vi "test12-RegisterMultipleStatesToOneState.vi"(8 "error in (no error)":errorcluster, 11 "TestCase in":refnum<class "testcase-CSMBroadcast.lvclass">) -> (0 "error out":errorcluster, 3 "TestCase out":refnum<class "testcase-CSMBroadcast.lvclass">)   [LabVIEW 2017, in "testcase-CSMBroadcast.lvclass"]
uses:
  testcase-CSMBroadcast.lvclass
  e86cc395-d992-44ca-a767-e0e34a6869d5.vi
  3bcad317-1b89-4687-aa9b-3ccbe7d60bbb.vi
  2694ea11-6498-4afa-8b48-991e2fec04f6.vi
  src/user.lib/_NEVSTOP/Communicable State Machine(CSM)/AdvanceAPI/CSM - Revert Arguments-Safe String.vi
  src/user.lib/_NEVSTOP/Communicable State Machine(CSM)/AdvanceAPI/CSM - Make String Arguments Safe.vi
  src/user.lib/_NEVSTOP/Communicable State Machine(CSM)/AdvanceAPI/CSM - Break Down Multiple States String.vi
  src/user.lib/_NEVSTOP/Communicable State Machine(CSM)/AdvanceAPI/CSM - Compact Multiple States.vi
  src/user.lib/_NEVSTOP/Communicable State Machine(CSM)/AdvanceAPI/CSM - Keywords.vi
  src/user.lib/_NEVSTOP/Communicable State Machine(CSM)/_Polymophic/CSM - Replace Marks in Messages.vi
  src/user.lib/_NEVSTOP/Communicable State Machine(CSM)/_Shared/Trim Single-line Text.vi
  src/user.lib/_NEVSTOP/Communicable State Machine(CSM)/AdvanceAPI/CSM - Set Module Attribute.vi
  src/user.lib/_NEVSTOP/Communicable State Machine(CSM)/AdvanceAPI/CSM - Get Module Attribute.vi
  <vilib>/addons/_JKI Toolkits/VI Tester/TestCase.llb/TestCase.lvclass
  src/user.lib/_NEVSTOP/Communicable State Machine(CSM)/Communicable State Machine.lvlib
  C:/Program Files (x86)/National Instruments/LabVIEW 2017/vi.lib/addons/_JKI Toolkits/VI Tester/TestCase.llb/TestCase.lvclass
panel:
  out "LoopCount":i32
  out "State History":string
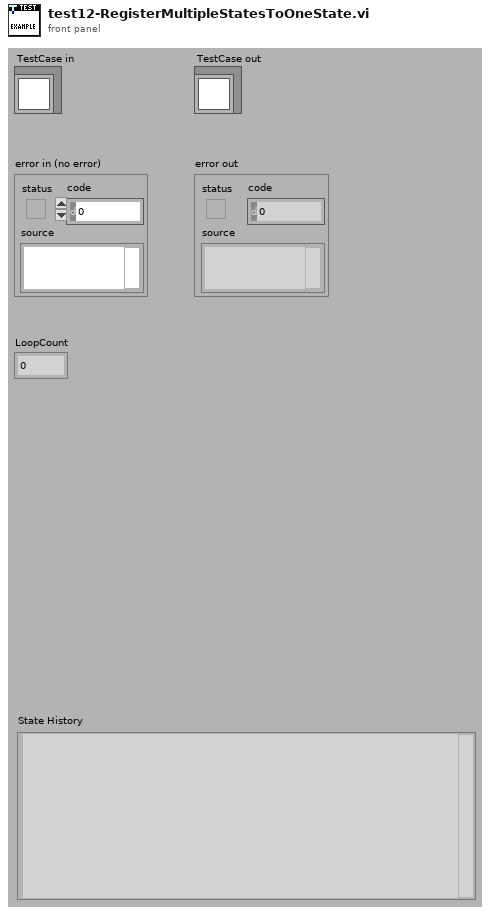
[diagram p1: front panel]
types:
  T1 = enum32{"Invalid", "Standard", "Closed", "Hidden", "Minimized", "Maximized"}
  T2 = enum32{"invalid app kind", "Development System", "Run Time System", "Student Edition", "Embedded LabVIEW", "Evaluation", "Custom"}
  T3 = typedef "Communicable State Machine.lvlib/_CSM_Response Source Message.ctl" = cluster{"‘State":string, "’Arguments":string, "’Error":errorcluster}
  T4 = cluster{"Current VI Reference":refnum<vi>, "Close Panel on Exit?":bool}
  T5 = cluster{"Core":cluster{"Current VI Reference":refnum<vi>, "Close Panel on Exit?":bool}, "Your Boolean data":bool, "Your string data":string, "TestData":i32}
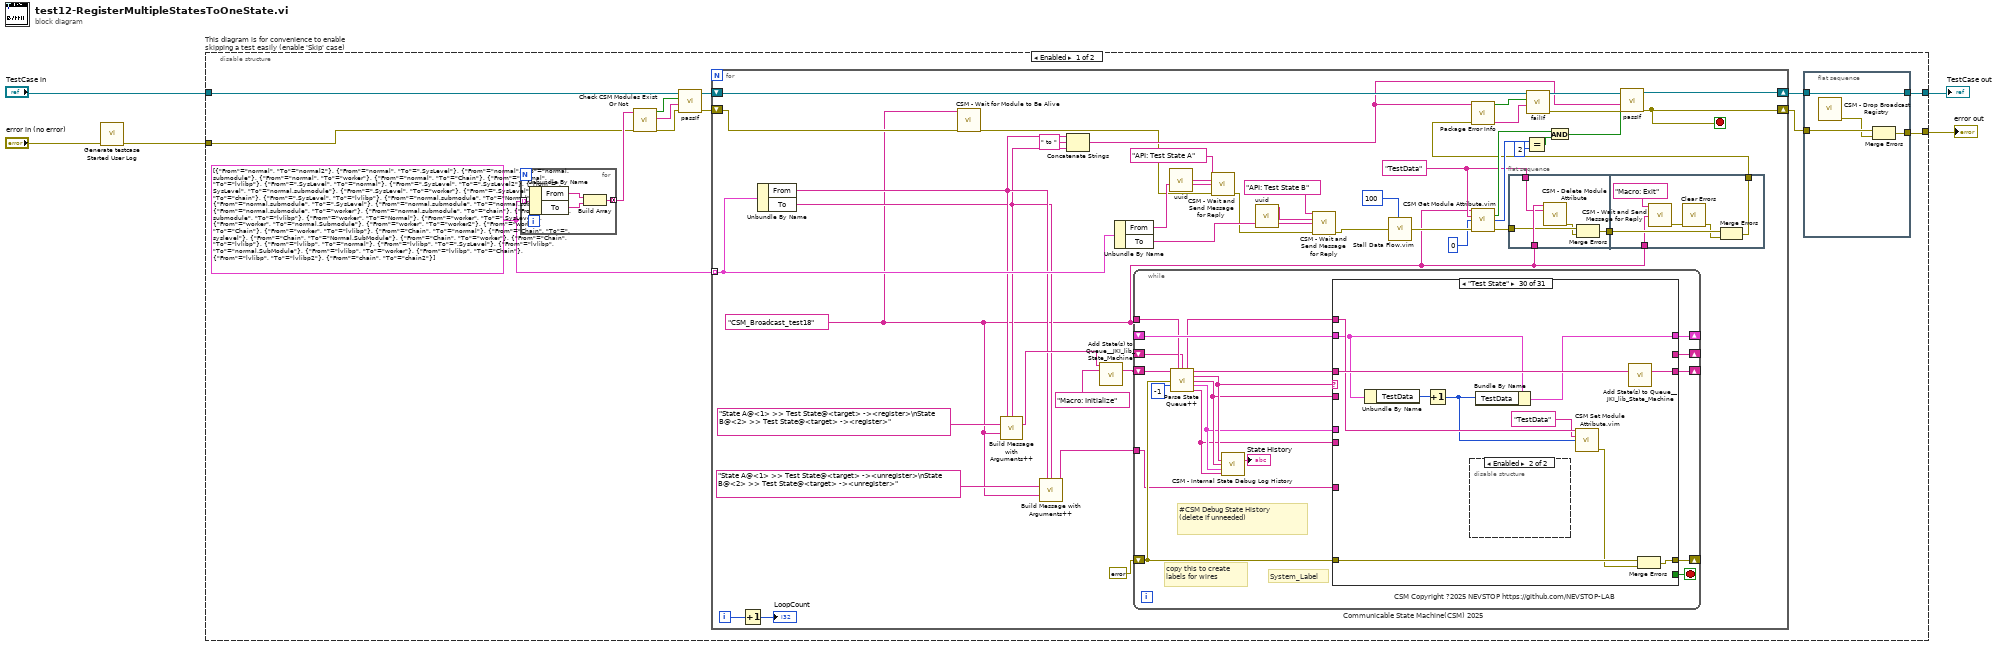
[diagram p0: block diagram]
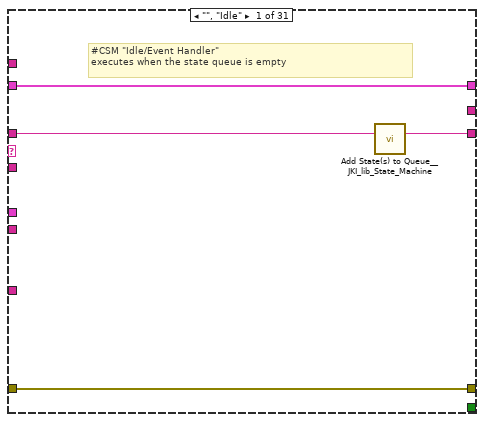
[diagram p2: hidden frame]
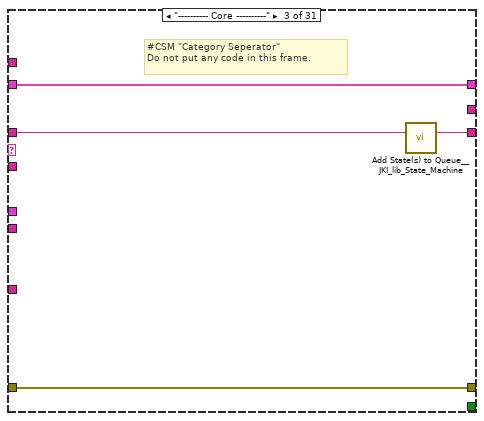
[diagram p4: hidden frame]
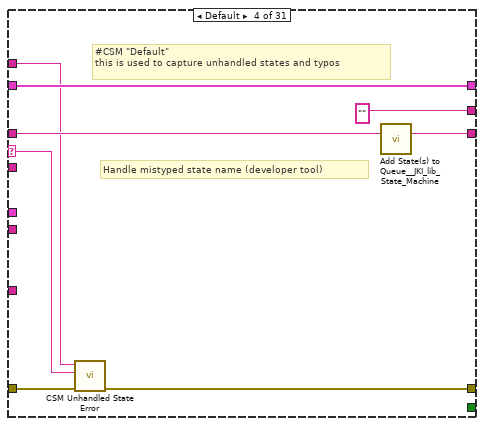
[diagram p5: hidden frame]
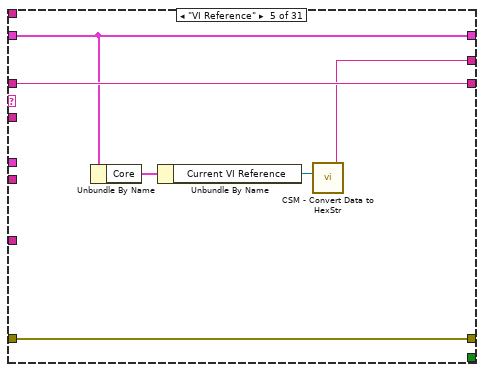
[diagram p6: hidden frame]
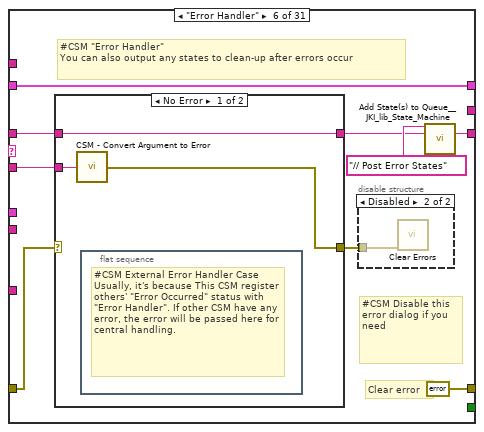
[diagram p7: hidden frame]
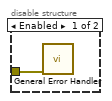
[diagram p8: hidden frame]
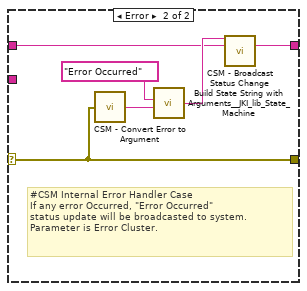
[diagram p9: hidden frame]
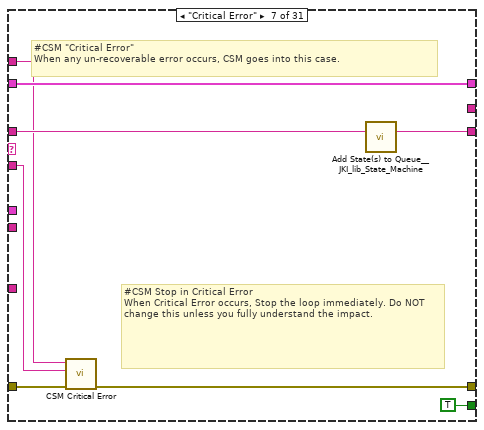
[diagram p10: hidden frame]
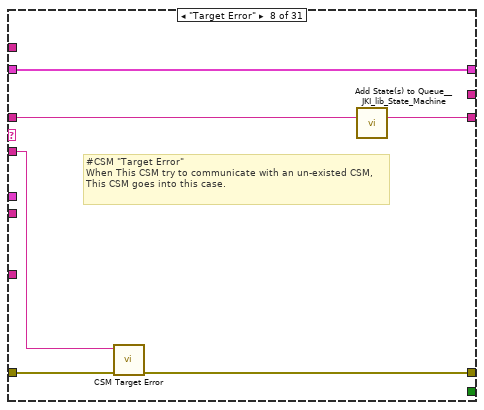
[diagram p11: hidden frame]
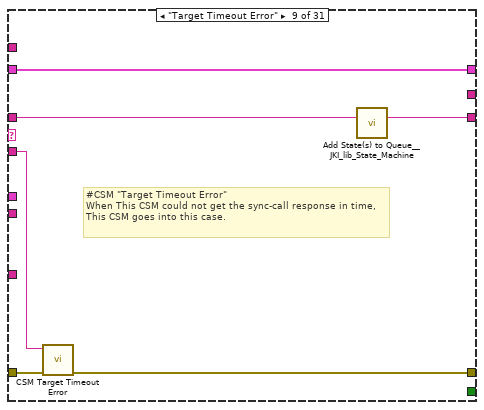
[diagram p12: hidden frame]
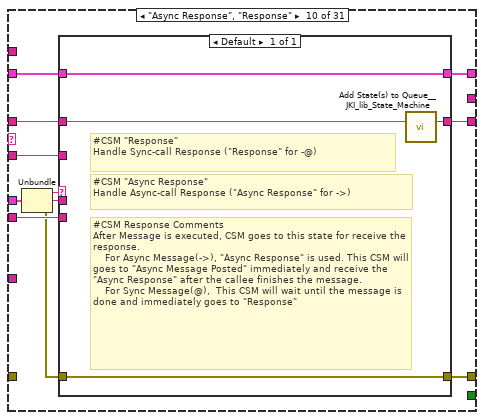
[diagram p13: hidden frame]
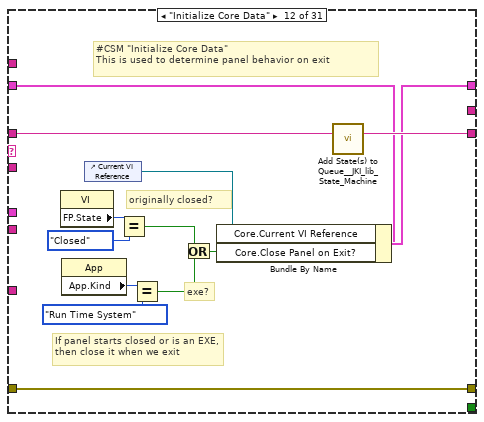
[diagram p15: hidden frame]
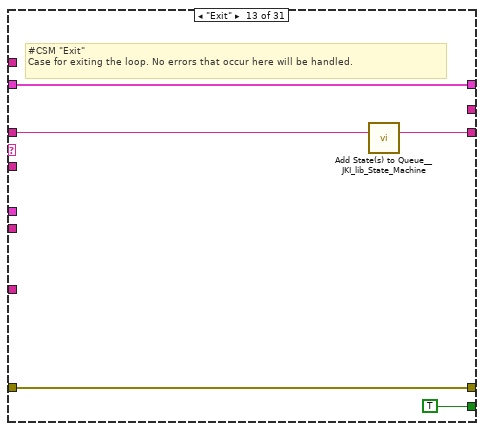
[diagram p16: hidden frame]
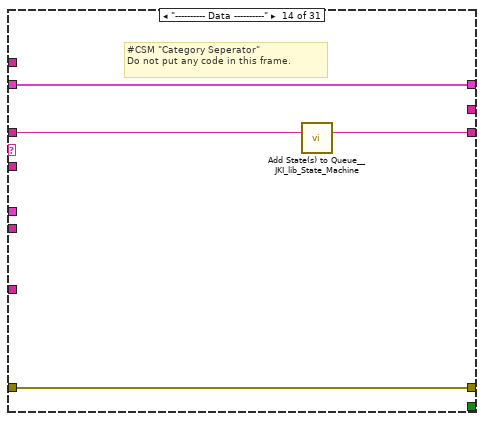
[diagram p17: hidden frame]
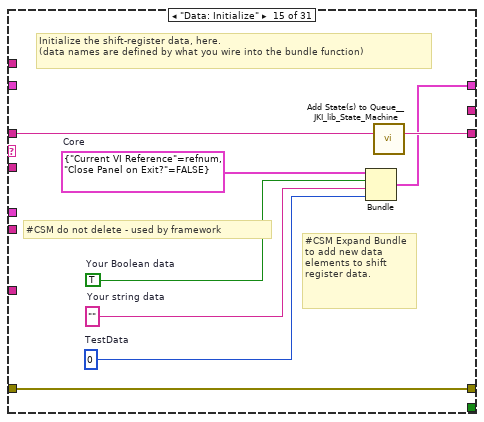
[diagram p18: hidden frame]
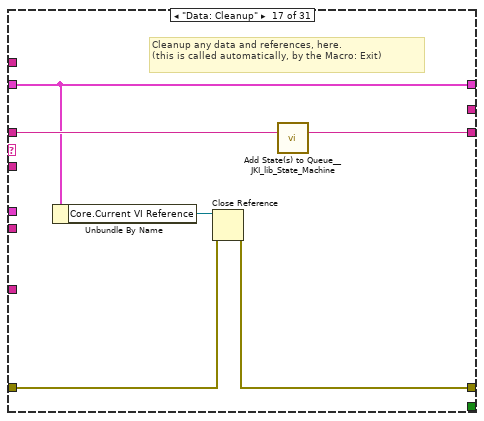
[diagram p20: hidden frame]
diagram:
  n1 = call "Generate testcase Started User Log.vi"("Error In"="error in (no error)") -> ("error out"=w1:errorcluster)  [unwired: 10 in]
  n2 = disable-structure "This diagram is for convenience to enable skipping a test easily (enable 'Skip' case)" shown="Enabled" {
    disable-tunnel: "TestCase in" -> [w9 w377]
    disable-tunnel: [w16 w375] -> w2
    disable-tunnel: [w15 w376] -> w4
    disable-tunnel: w1 -> [w6 w374]
    frame Enabled {
      w10 = cluster{"From":string, "To":string}[] [{"From"="normal", "To"="normal2"}, {"From"="normal", "To"=".SysLevel"}, {"From"="normal", "To"="normal.submodule"}, {"From"="normal", "To"="worker"}, {"From"="normal", "To"="Chain"}, {"From"="normal", "To"="lvlibp"}, {"From"=".SysLevel", "To"="normal"}, {"From"=".SysLevel", "To"=".SysLevel2"}, {"From"=".SysLevel", "To"="normal.submodule"}, {"From"=".SysLevel", "To"="worker"}, {"From"=".SysLevel", "To"="chain"}, {"From"=".SysLevel", "To"="lvlibp"}, {"From"="normal.submodule", "To"="Normal"}, {"From"="normal.submodule", "To"=".SysLevel"}, {"From"="normal.submodule", "To"="normal.submodule2"}, {"From"="normal.submodule", "To"="worker"}, {"From"="normal.submodule", "To"="chain"}, {"From"="normal.submodule", "To"="lvlibp"}, {"From"="worker", "To"="Normal"}, {"From"="worker", "To"=".SysLevel"}, {"From"="worker", "To"="normal.Submodule"}, {"From"="worker", "To"="worker2"}, {"From"="worker", "To"="Chain"}, {"From"="worker", "To"="lvlibp"}, {"From"="Chain", "To"="normal"}, {"From"="Chain", "To"=".syslevel"}, {"From"="Chain", "To"="Normal.SubModule"}, {"From"="Chain", "To"="worker"}, {"From"="Chain", "To"="lvlibp"}, {"From"="lvlibp", "To"="normal"}, {"From"="lvlibp", "To"=".SysLevel"}, {"From"="lvlibp", "To"="normal.SubModule"}, {"From"="lvlibp", "To"="worker"}, {"From"="lvlibp", "To"="Chain"}, {"From"="lvlibp", "To"="lvlibp2"}, {"From"="chain", "To"="chain2"}]
      n3 = for {
        tunnel: w10 -> [w22] mode=indexing
        tunnel: [w19] -> w13 mode=concatenating
        n4 = Unbundle By Name(w22) -> ("From"=w21:string, "To"=w20:string)
        n5 = Build Array(w21, w20) -> (w19:string[])
      }
      n6 = call "Check CSM Modules Exist Or Not.vi"("error in"=w6, "CSM names in"=w13) -> ("error out"=w11:errorcluster, "Debug string"=w12:string, "All Modules Exist?"=w14:bool)  [unwired: 7 in]
      n7 = call-dynamic "passIf.vi"("error in (no error)"=w11, "message (\"\")"=w12, "pass"=w14, "TestCase in"=w9) -> ("error out"=w7:errorcluster, "TestCase out"=w8:refnum<class "testcase-CSMBroadcast.lvclass">)  [unwired: 6 in]
      n8 = for {
        tunnel: w10 -> [w61] mode=indexing
        shift-right: [w48] -> w18
        shift-left: w8 -> [w39]
        shift-right: [w47] -> w17
        shift-left: w7 -> [w31]
        i -> [w46]
        stop <- w47 stop-if-true
        w50 = "TestData" ("Attribute")
        w29 = "CSM_Broadcast_test18" ("Name (\"\" to Use UUID)")
        n9 = Increment(x=w46) -> (x+1=→"LoopCount":i32)
        n10 = Unbundle By Name(w61) -> ("From"=w35:string, "To"=w34:string)
        n11 = call "CSM - Wait for Module to Be Alive.vi"("CSM Name"=w29, "error in (no error)"=w31) -> ("error out"=w30:errorcluster)  [unwired: 11 in, 2 out]
        n12 = call-poly "Build Message with Arguments++.vi"("States With Replace Token"="State A@<1> >> Test State@<target> -><register>\nState B@<2> >> Test State@<target> -><register>" ("Init State(\"Macro: Initialize\")"), "<target>"=w29, "<1>"=w35, "<2>"=w34) -> ("States"=w59:string)  [unwired: 11 in]
        n13 = call-poly "Build Message with Arguments++.vi"("States With Replace Token"="State A@<1> >> Test State@<target> -><unregister>\nState B@<2> >> Test State@<target> -><unregister>" ("Init State(\"Macro: Initialize\")"), "<target>"=w29, "<1>"=w35, "<2>"=w34) -> ("States"=w57:string)  [unwired: 11 in]
        n14 = Concatenate Strings(w35, " to " ("string"), w34) -> (w32:string)
        n15 = call <vilib>:"Add State(s) to Queue__JKI_lib_State_Machine.vi"("State(s) in Front (\"\")"=w59, "State(s) in (\"\")"="Macro: Initialize" ("Init State(\"Macro: Initialize\")")) -> ("States Out"=w62:string)  [unwired: 13 in]
        n16 = Unbundle By Name(w61) -> ("From"=w68:string, "To"=w67:string)
        n17 = while "Communicable State Machine(CSM) 2025" {
          shift-right: [w95] -> _
          shift-left: _ -> [w94]
          shift-right: [w98] -> _
          shift-left: errorcluster {"status"=FALSE, "code"=0, "source"=""} ("error out") -> [w93]
          shift-right: [w97] -> _
          shift-left: w62 -> [w99]
          tunnel: w29 -> [w91]
          shift-right: [w92] -> _
          shift-left: _ -> [w85]
          tunnel: w57 -> [w82]
          stop <- w96 stop-if-true
          # "#CSM Debug State History\n(delete if unneeded)"
          # "copy this to create labels for wires"
          # "System_Label"
          # "CSM Copyright ?2025 NEVSTOP https://github.com/NEVSTOP-LAB"
          n18 = call "Parse State Queue++.vi"("State Queue"=w99, "Name (\"\" to Use UUID)"=w91, "Response Arguments"=w85, "Previous Error"=w93, "Dequeue (1 ms)"=-1 ("Timeout")) -> ("Name Used"=w86:string, "Remaining States"=w100:string, "Current State"=w90:string, "Arguments"=w89:string, "Additional Information"=w88:T3, "Source CSM"=w87:string)  [unwired: 5 in]
          n19 = call "CSM - Internal State Debug Log History.vi"("State"=w90, "Arguments (\"\")"=w89, ">> Response Source Message >>"=w88, "Source (\"\")"=w87) -> ("Debug Log"=→"State History":string)  [unwired: 11 in]
          n20 = case shown="\"Test State\"" w90 {
            selector: w90 -> [_ _ _ w114 _ _ _ _ _ _ _ _ _ _ _ _ _ _ _ _ _ _ _ _ _ _ _ _ _ _ _]
            tunnel: w100 -> [w101 w106 w111 w118 w124 w130 w151 w157 w163 w171 w182 w196 w201 w205 w213 w215 w222 w226 w230 w236 w251 w320 w325 w333 w335 w339 w344 w351 w355 w366 w373]
            tunnel: w89 -> [_ _ _ _ _ w129 w147 w156 w161 w170 _ _ _ _ _ _ _ _ _ w231 w245 _ _ _ _ _ w342 _ _ _ _]
            tunnel: w94 -> [w102 w105 w108 w116 w123 w133 w152 w158 w164 w173 w181 w189 w199 w202 _ w214 w217 w223 w228 w234 w247 w317 w322 w330 w334 w338 w343 w348 w352 w358 w370]
            tunnel: [w103 w107 w109 w112 w125 errorcluster {"status"=FALSE, "code"=0, "source"=""} ("error out") w148 w154 w160 w176 w183 w193 w198 w203 w210 w216 w218 w224 w227 w232 w248 w318 w323 w331 w336 w340 w345 w349 w353 w360 w371] -> w98
            tunnel: w93 -> [w103 w107 w109 w119 w125 w131 w153 w155 w162 _ w183 w193 w198 w203 w210 w216 w219 w224 w227 w233 w249 w318 w323 w331 w336 w340 w345 w349 w353 w364 w371]
            tunnel: [w104 w106 w110 w117 w124 w126 w150 w159 w165 w172 w182 w195 w200 w204 w212 w215 w221 w225 w229 w235 w250 w319 w324 w332 w335 w339 w344 w350 w354 w365 w372] -> w97
            tunnel: [_ _ _ _ _ _ TRUE _ _ _ _ _ TRUE _ _ _ _ _ _ _ _ _ _ _ _ _ _ _ _ _ _] -> w96
            tunnel: [w102 w105 w108 w116 w123 w133 w152 w158 w164 w174 w181 w194 w199 w202 w211 w214 w217 w223 w228 w234 w247 w317 w322 w330 w334 w338 w343 w348 w352 w362 w370] -> w95
            tunnel: w87 -> [_ _ _ _ _ _ _ _ _ w168 _ _ _ _ _ _ _ _ _ _ _ _ _ _ _ _ _ _ _ _ _]
            tunnel: w88 -> [_ _ _ _ _ _ _ _ _ w175 _ _ _ _ _ _ _ _ _ _ _ _ _ _ _ _ _ _ _ _ _]
            tunnel: [_ _ _ "" w120 _ _ _ _ _ _ _ _ _ _ _ _ _ _ _ _ _ _ _ _ "API1 Response" w341 _ _ _ _] -> w92
            tunnel: w86 -> [_ _ _ w113 _ _ w146 _ _ _ _ _ _ _ _ _ _ _ _ _ _ _ _ _ _ _ _ _ _ w361 _]
            tunnel: w82 -> [_ _ _ _ _ _ _ _ _ _ _ _ _ _ _ _ _ _ _ _ _ _ _ w326 _ _ _ _ _ _ _]
            frame "", "Idle" {
              # "#CSM \"Idle/Event Handler\"\nexecutes when the state queue is empty"
              n21 = call <vilib>:"Add State(s) to Queue__JKI_lib_State_Machine.vi"("State(s) in (\"\")"=w101) -> ("States Out"=w104:string)  [unwired: 14 in]
            }
            frame "CSM Documentation" {
              # "#CSM README FIRST\n\nCommunicable State Machine(CSM) is a LabVIEW application framework that builds upon JKI State Machine(JKISM). It follows the pattern of JKISM and extends the keywords to describe message communication between modules, including concepts such as Sync-Message, Async-Message, Subscription/Unsubscription of status - essential elements for creating reusable code modules. For more information, please visit the CSM wiki: https://nevstop-lab.github.io/CSM-Wiki/\n\nFor instructions on JKI State Machine, visit: http://jki.net/state-machine/\nFor information about CSM, visit: https://github.com/NEVSTOP-LAB"
              # "#CSM \"Documentation\"\nCase for holding CSM Documenation"
            }
            frame "---------- Core ----------" {
              # "#CSM \"Category Seperator\"\nDo not put any code in this frame."
              n22 = call <vilib>:"Add State(s) to Queue__JKI_lib_State_Machine.vi"("State(s) in (\"\")"=w111) -> ("States Out"=w110:string)  [unwired: 14 in]
            }
            frame Default {
              # "#CSM \"Default\"\nthis is used to capture unhandled states and typos"
              # "Handle mistyped state name (developer tool)"
              n23 = call "CSM Unhandled State Error.vi"("error in (no error)"=w119, "Undefined State"=w114, "CSM Name"=w113) -> ("error out"=w112:errorcluster)  [unwired: 8 in]
              n24 = call <vilib>:"Add State(s) to Queue__JKI_lib_State_Machine.vi"("State(s) in (\"\")"=w118) -> ("States Out"=w117:string)  [unwired: 14 in]
            }
            frame "VI Reference" {
              n25 = Unbundle By Name(w123) -> ("Core"=w122:T4)
              n26 = Unbundle By Name(w122) -> ("Current VI Reference"=w121:refnum<vi>)
              n27 = call "CSM - Convert Data to HexStr.vi"("Variant"=w121) -> ("HEX String (0-9,A-F)"=w120:string)  [unwired: 8 in]
            }
            frame "Error Handler" {
              # "#CSM Disable this error dialog if you need"
              # "#CSM \"Error Handler\"\nYou can also output any states to clean-up after errors occur"
              # "Clear error"
              n28 = case shown="No Error" w131 {
                selector: w131 -> [_ w140]
                tunnel: [w139 w142] -> w127
                tunnel: w130 -> [w139 w141]
                tunnel: w129 -> [w138 _]
                tunnel: [w137 w140] -> w132
                frame No Error {
                  n29 = call "CSM - Convert Argument to Error.vi"("Argument"=w138) -> ("Error"=w137:errorcluster)  [unwired: 4 in]
                  n30 = flat-sequence {
                    frame #0 {
                      # "#CSM External Error Handler Case\nUsually, it's because This CSM register others' \"Error Occurred\" status with \"Error Handler\". If other CSM have any error, the error will be passed here for central handling."
                    }
                  }
                }
                frame Error {
                  # "#CSM Internal Error Handler Case \nIf any error Occurred, \"Error Occurred\" \nstatus update will be broadcasted to system.\nParameter is Error Cluster."
                  n31 = call "CSM - Convert Error to Argument.vi"("Error"=w140) -> ("Argument"=w144:string)  [unwired: 4 in]
                  n32 = call <vilib>:"Build State String with Arguments__JKI_lib_State_Machine.vi"("Arguments (\"\")"=w144, "State"="Error Occurred" ("Status with Arguments")) -> ("State with Arguments"=w143:string)  [unwired: 4 in]
                  n33 = call "CSM - Broadcast Status Change.vi"("Status With Arguments"=w143, "State Queue"=w141) -> ("Remaining States"=w142:string)  [unwired: 13 in]
                }
              }
              n34 = disable-structure shown="Disabled" {
                disable-tunnel: w132 -> [w135 w136]
                frame Enabled {
                  n35 = call <vilib>:"General Error Handler.vi"("error in (no error)"=w135) -> ()  [unwired: 10 in, 5 out]
                }
                frame Disabled {
                  n36 = call <vilib>:"Clear Errors.vi"("error in (no error)"=w136) -> ()  [unwired: 5 in, 2 out]
                }
              }
              n37 = call <vilib>:"Add State(s) to Queue__JKI_lib_State_Machine.vi"("State(s) in Front (\"\")"="// Post Error States", "State(s) in (\"\")"=w127) -> ("States Out"=w126:string)  [unwired: 13 in]
            }
            frame "Critical Error" {
              # "#CSM Stop in Critical Error\nWhen Critical Error occurs, Stop the loop immediately. Do NOT change this unless you fully understand the impact."
              # "#CSM \"Critical Error\"\nWhen any un-recoverable error occurs, CSM goes into this case."
              n38 = call "CSM Critical Error.vi"("error in (no error)"=w153, "Arugments (As Reason)"=w147, "CSM Name"=w146) -> ("error out"=w148:errorcluster)  [unwired: 8 in]
              n39 = call <vilib>:"Add State(s) to Queue__JKI_lib_State_Machine.vi"("State(s) in (\"\")"=w151) -> ("States Out"=w150:string)  [unwired: 14 in]
            }
            frame "Target Error" {
              # "#CSM \"Target Error\"\nWhen This CSM try to communicate with an un-existed CSM, This CSM goes into this case."
              n40 = call "CSM Target Error.vi"("error in (no error)"=w155, "Arguments (As CSM Name)"=w156) -> ("error out"=w154:errorcluster)  [unwired: 9 in]
              n41 = call <vilib>:"Add State(s) to Queue__JKI_lib_State_Machine.vi"("State(s) in (\"\")"=w157) -> ("States Out"=w159:string)  [unwired: 14 in]
            }
            frame "Target Timeout Error" {
              # "#CSM \"Target Timeout Error\"\nWhen This CSM could not get the sync-call response in time, This CSM goes into this case."
              n42 = call "CSM Target Timeout Error.vi"("error in (no error)"=w162, "Arguments (As CSM Name)"=w161) -> ("error out"=w160:errorcluster)  [unwired: 9 in]
              n43 = call <vilib>:"Add State(s) to Queue__JKI_lib_State_Machine.vi"("State(s) in (\"\")"=w163) -> ("States Out"=w165:string)  [unwired: 14 in]
            }
            frame "Async Response", "Response" {
              n44 = Unbundle(w175) -> ("‘State"=w169:string, "’Arguments"=w167:string, "’Error"=w166:errorcluster)
              n45 = case shown="Default" w169 {
                tunnel: [w180] -> w176
                tunnel: w166 -> [w180]
                tunnel: [w179] -> w174
                tunnel: w173 -> [w179]
                tunnel: [w177] -> w172
                tunnel: w171 -> [w178]
                tunnel: w170 -> [_]
                tunnel: w168 -> [_]
                tunnel: w167 -> [_]
                frame Default {
                  # "#CSM Response Comments\nAfter Message is executed, CSM goes to this state for receive the response.\n    For Async Message(->), \"Async Response\" is used. This CSM will goes to \"Async Message Posted\" immediately and receive the \"Async Response\" after the callee finishes the message.\n    For Sync Message(@),  This CSM will wait until the message is done and immediately goes to \"Response\""
                  # "#CSM \"Async Response\"\nHandle Async-call Response (\"Async Response\" for ->)"
                  # "#CSM \"Response\"\nHandle Sync-call Response (\"Response\" for -@)"
                  n46 = call <vilib>:"Add State(s) to Queue__JKI_lib_State_Machine.vi"("State(s) in (\"\")"=w178) -> ("States Out"=w177:string)  [unwired: 14 in]
                }
              }
            }
            frame "Async Message Posted" {
              # "#CSM \"Async Message Posted\"\nAfter Async Message is posted (-> or ->| ), CSM goes to this state for post-action.\nYou can use Argument - State to tell which Async Message is called."
            }
            frame "Initialize Core Data" {
              # "#CSM \"Initialize Core Data\"\nThis is used to determine panel behavior on exit"
              # "originally closed?"
              # "exe?"
              # "If panel starts closed or is an EXE, then close it when we exit"
              n47 = property class="VI"() -> ("FP.State"=w186:T1)  [unwired: 2 in, 2 out]
              n48 = property class="App"() -> ("App.Kind"=w192:T2)  [unwired: 2 in, 2 out]
              n49 = control-ref of="Current VI Reference"() -> (w187:refnum<vi>)
              n50 = Equal?(x=w186, y=T1."Closed" ("Front Panel Window:State")) -> (x = y?=w184:bool)
              n51 = Equal?(x=w192, y=T2."Run Time System" ("Application:Kind")) -> (x = y?=w190:bool)
              n52 = Or(x=w184, y=w190) -> (x .or. y?=w188:bool)
              n53 = Bundle By Name(cluster=w189, "Core.Current VI Reference"=w187, "Core.Close Panel on Exit?"=w188) -> (w194:T5)
              n54 = call <vilib>:"Add State(s) to Queue__JKI_lib_State_Machine.vi"("State(s) in (\"\")"=w196) -> ("States Out"=w195:string)  [unwired: 14 in]
            }
            frame "Exit" {
              # "#CSM \"Exit\"\nCase for exiting the loop. No errors that occur here will be handled."
              n55 = call <vilib>:"Add State(s) to Queue__JKI_lib_State_Machine.vi"("State(s) in (\"\")"=w201) -> ("States Out"=w200:string)  [unwired: 14 in]
            }
            frame "---------- Data ----------" {
              # "#CSM \"Category Seperator\"\nDo not put any code in this frame."
              n56 = call <vilib>:"Add State(s) to Queue__JKI_lib_State_Machine.vi"("State(s) in (\"\")"=w205) -> ("States Out"=w204:string)  [unwired: 14 in]
            }
            frame "Data: Initialize" {
              w206 = 0  # TestData
              w207 = T4 {"Current VI Reference"=refnum, "Close Panel on Exit?"=FALSE}  # Core
              w209 = TRUE  # Your Boolean data
              w208 = ""  # Your string data
              # "#CSM do not delete - used by framework"
              # "#CSM Expand Bundle to add new data elements to shift register data."
              # "Initialize the shift-register data, here.\n(data names are defined by what you wire into the bundle function)"
              n57 = Bundle("Core"=w207, "Your Boolean data"=w209, "Your string data"=w208, "TestData"=w206) -> (w211:T5)  [unwired: 1 in]
              n58 = call <vilib>:"Add State(s) to Queue__JKI_lib_State_Machine.vi"("State(s) in (\"\")"=w213) -> ("States Out"=w212:string)  [unwired: 14 in]
            }
            frame "Data: Update Indicators" {
            }
            frame "Data: Cleanup" {
              # "Cleanup any data and references, here.\n(this is called automatically, by the Macro: Exit)"
              n59 = Unbundle By Name(w217) -> ("Core.Current VI Reference"=w220:refnum<vi>)
              n60 = Close Reference(reference=w220, error in (no error)=w219) -> (error out=w218:errorcluster)
              n61 = call <vilib>:"Add State(s) to Queue__JKI_lib_State_Machine.vi"("State(s) in (\"\")"=w222) -> ("States Out"=w221:string)  [unwired: 14 in]
            }
            frame "---------- UI ----------" {
              # "#CSM \"Category Seperator\"\nDo not put any code in this frame."
              n62 = call <vilib>:"Add State(s) to Queue__JKI_lib_State_Machine.vi"("State(s) in (\"\")"=w226) -> ("States Out"=w225:string)  [unwired: 14 in]
            }
            frame "UI: Initialize" {
              # "#CSM \"UI: Initialize\"\nInitialize the User Interface, here.\n(this is called automatically, by the Macro: Init)"
              n63 = call <vilib>:"Add State(s) to Queue__JKI_lib_State_Machine.vi"("State(s) in (\"\")"=w230) -> ("States Out"=w229:string)  [unwired: 14 in]
            }
            frame "UI: Cursor Set" {
              # "#CSM \"UI: Cursor Set\"\nSet and Unset Cursor Busy.\n(Usage: \"UI: Cursor Set >> Busy|Idle\")"
              # "Argument"
              n64 = disable-structure shown="TARGET_TYPE!=Windows" {
                disable-tunnel: w233 -> [w239 w244]
                disable-tunnel: [w238 w244] -> w232
                disable-tunnel: w231 -> [w237 _]
                frame condition #0 (active) {
                  n65 = case shown="\"Idle\", Default" w237 {
                    tunnel: w239 -> [w241 w243]
                    tunnel: [w240 w242] -> w238
                    frame "Idle", Default {
                      n66 = call <vilib>:"Unset Busy.vi"("error in (no error)"=w241) -> ("error out"=w240:errorcluster)  [unwired: 10 in]
                    }
                    frame "Busy" {
                      n67 = call <vilib>:"Set Busy.vi"("error in (no error)"=w243) -> ("error out"=w242:errorcluster)  [unwired: 9 in, 1 out]
                    }
                  }
                }
                frame condition #1 {
                }
              }
              n68 = call <vilib>:"Add State(s) to Queue__JKI_lib_State_Machine.vi"("State(s) in (\"\")"=w236) -> ("States Out"=w235:string)  [unwired: 14 in]
            }
            frame "UI: Front Panel State" {
              # "#CSM \"UI: Front Panel State\"\nSet Front Panel Open or Closed\n(Usage: \"UI: Front Panel State >> Open|Close\")"
              # "Argument"
              n69 = Unbundle By Name(w247) -> ("Core.Current VI Reference"=w246:refnum<vi>)
              n70 = call <vilib>:"Add State(s) to Queue__JKI_lib_State_Machine.vi"("State(s) in (\"\")"=w251) -> ("States Out"=w250:string)  [unwired: 14 in]
              n71 = case shown="\"Close\", \"Closed\"" w245 {
                tunnel: w249 -> [w257 w272 w283 w296 w309]
                tunnel: [w259 w273 w285 w298 w311] -> w248
                tunnel: w246 -> [w258 w270 w284 w297 w310]
                frame "Open", "Standard", Default {
                  w252 = T1."Standard" ("State")
                  n72 = property class="VI"(reference=w258, error in=w257) -> (reference out=w255:refnum<vi>, error out=w256:errorcluster, "FP.State"=w254:T1)
                  n73 = Not Equal?(x=w254, y=w252) -> (x != y?=w253:bool)
                  n74 = case shown="True" w253 {
                    tunnel: [w263 w265] -> w259
                    tunnel: w256 -> [w262 w265]
                    tunnel: w255 -> [w261 _]
                    tunnel: w252 -> [w260 _]
                    frame True {
                      n75 = invoke class="VI" method="FP.Open"(reference=w261, error in=w262, "Activate"=TRUE, "State"=w260) -> (error out=w263:errorcluster)  [unwired: 1 in, 4 out]
                    }
                    frame False {
                    }
                  }
                }
                frame "Close", "Closed" {
                  n76 = property class="VI"(reference=w270, error in=w272) -> (reference out=w269:refnum<vi>, error out=w271:errorcluster, "FP.State"=w267:T1)
                  n77 = Not Equal?(x=w267, y=T1."Closed" ("Front Panel Window:State")) -> (x != y?=w266:bool)
                  n78 = case shown="False" w266 {
                    tunnel: [w274 w277] -> w273
                    tunnel: w271 -> [w274 w276]
                    tunnel: w269 -> [_ w275]
                    frame False {
                    }
                    frame True {
                      n79 = invoke class="VI" method="FP.Close"(reference=w275, error in=w276) -> (error out=w277:errorcluster)  [unwired: 1 in, 2 out]
                    }
                  }
                }
                frame "Hidden", "Hide" {
                  w278 = T1."Hidden" ("State")
                  n80 = property class="VI"(reference=w284, error in=w283) -> (reference out=w281:refnum<vi>, error out=w282:errorcluster, "FP.State"=w280:T1)
                  n81 = Not Equal?(x=w280, y=w278) -> (x != y?=w279:bool)
                  n82 = case shown="True" w279 {
                    tunnel: [w289 w290] -> w285
                    tunnel: w282 -> [w288 w290]
                    tunnel: w281 -> [w287 _]
                    tunnel: w278 -> [w286 _]
                    frame True {
                      n83 = invoke class="VI" method="FP.Open"(reference=w287, error in=w288, "State"=w286) -> (error out=w289:errorcluster)  [unwired: 2 in, 4 out]
                    }
                    frame False {
                    }
                  }
                }
                frame "Minimize", "Minimized" {
                  w291 = T1."Minimized" ("State")
                  n84 = property class="VI"(reference=w297, error in=w296) -> (reference out=w294:refnum<vi>, error out=w295:errorcluster, "FP.State"=w293:T1)
                  n85 = Not Equal?(x=w293, y=w291) -> (x != y?=w292:bool)
                  n86 = case shown="True" w292 {
                    tunnel: [w302 w303] -> w298
                    tunnel: w295 -> [w301 w303]
                    tunnel: w294 -> [w300 _]
                    tunnel: w291 -> [w299 _]
                    frame True {
                      n87 = invoke class="VI" method="FP.Open"(reference=w300, error in=w301, "State"=w299) -> (error out=w302:errorcluster)  [unwired: 2 in, 4 out]
                    }
                    frame False {
                    }
                  }
                }
                frame "Maximize", "Maximized" {
                  w304 = T1."Maximized" ("State")
                  n88 = property class="VI"(reference=w310, error in=w309) -> (reference out=w307:refnum<vi>, error out=w308:errorcluster, "FP.State"=w306:T1)
                  n89 = Not Equal?(x=w306, y=w304) -> (x != y?=w305:bool)
                  n90 = case shown="True" w305 {
                    tunnel: [w315 w316] -> w311
                    tunnel: w308 -> [w314 w316]
                    tunnel: w307 -> [w313 _]
                    tunnel: w304 -> [w312 _]
                    frame True {
                      n91 = invoke class="VI" method="FP.Open"(reference=w313, error in=w314, "State"=w312) -> (error out=w315:errorcluster)  [unwired: 2 in, 4 out]
                    }
                    frame False {
                    }
                  }
                }
              }
            }
            frame "---------- Macro ----------" {
              # "#CSM \"Category Seperator\"\nDo not put any code in this frame."
              n92 = call <vilib>:"Add State(s) to Queue__JKI_lib_State_Machine.vi"("State(s) in (\"\")"=w320) -> ("States Out"=w319:string)  [unwired: 14 in]
            }
            frame "Macro: Initialize" {
              # "#CSM \"Macro: Initialize\"\nInitialization Macro (This is called once, when the VI starts)"
              n93 = call <vilib>:"Add State(s) to Queue__JKI_lib_State_Machine.vi"("State(s) in Front (\"\")"="Data: Initialize\nInitialize Core Data\nData: Update Indicators", "State(s) in (\"\")"=w325) -> ("States Out"=w324:string)  [unwired: 13 in]
            }
            frame "Macro: Exit" {
              # "#CSM \"Macro: Exit\"\nExit Macro (This is called once, when the VI exits)"
              n94 = call <vilib>:"Add State(s) to Queue__JKI_lib_State_Machine.vi"("State(s) in Front (\"\")"="//Exit Sub-Modules ", "State(s) in (\"\")"=w326, "State(s) at Back (\"\")"="Data: Cleanup\nExit") -> ("States Out"=w328:string)  [unwired: 12 in]
              n95 = call <vilib>:"Add State(s) to Queue__JKI_lib_State_Machine.vi"("State(s) in Front (\"\")"=w328, "State(s) in (\"\")"=w333) -> ("States Out"=w332:string)  [unwired: 13 in]
            }
            frame "---------- API ----------" {
              # "#CSM \"Category Seperator\"\nDo not put any code in this frame."
            }
            frame "API: API1" {
              # "#CSM API Example\nCopy/Rename this case for your own API"
              # "#CSM Response\nConnect this to return the response of your API"
              # "#CSM >> Msg/Rep's CSM >>\nIf you need to tell who triggered this state , use this string. If it's this case itself, this string is \"\"."
              # "#CSM >> Arguments >>\nDeal with the parameter if any"
            }
            frame "API: API2" {
              # "#CSM API Example\nCopy/Rename this case for your own API"
              # "unpack Hex String  to Variant\nif complex parameter is needed."
              n96 = call "CSM - Convert HexStr to Data.vi"("HEX String"=w342) -> ()  [unwired: 7 in, 2 out]
              n97 = disable-structure shown="Disabled" {
                disable-tunnel: [w346 "API2 Response"] -> w341
                frame Disabled {
                  # "pack variant to hexstr \nif complex response is needed."
                  # "complex Response"
                  n98 = call "CSM - Convert Data to HexStr.vi"() -> ("HEX String (0-9,A-F)"=w346:string)  [unwired: 9 in]
                }
                frame Enabled {
                }
              }
            }
            frame "---------- Action ----------" {
              # "#CSM \"Category Seperator\"\nDo not put any code in this frame."
              n99 = call <vilib>:"Add State(s) to Queue__JKI_lib_State_Machine.vi"("State(s) in (\"\")"=w351) -> ("States Out"=w350:string)  [unwired: 14 in]
            }
            frame "Action: action1" {
              # "#CSM \"Internal State\"\nThis category is used for holding internal states"
              n100 = call <vilib>:"Add State(s) to Queue__JKI_lib_State_Machine.vi"("State(s) in (\"\")"=w355) -> ("States Out"=w354:string)  [unwired: 14 in]
            }
            frame "Test State" {
              n101 = Unbundle By Name(w358) -> ("TestData"=w363:i32)
              n102 = Increment(x=w363) -> (x+1=w356:i32)
              n103 = disable-structure shown="Enabled" {
                frame Disabled {
                  n104 = feedback #1(0 ("y")) -> (w368:i32)
                  n105 = Increment(x=w368) -> (x+1=w367:i32)
                  n106 = feedback-in #1(w367) -> ()
                }
                frame Enabled {
                }
              }
              n107 = Bundle By Name(cluster=w358, "TestData"=w356) -> (w362:T5)
              n108 = call "CSM Set Module Attribute.vim"("CSM Name"=w361, "Attribute"="TestData", "Value"=w356) -> ("error out"=w359:errorcluster)  [unwired: 9 in, 3 out]
              n109 = call <vilib>:"Add State(s) to Queue__JKI_lib_State_Machine.vi"("State(s) in (\"\")"=w366) -> ("States Out"=w365:string)  [unwired: 14 in]
              n110 = Merge Errors(w364, w359) -> (w360:errorcluster)
            }
            frame "Action: action2" {
              # "#CSM \"Internal State\"\nThis category is used for holding internal states"
              n111 = call <vilib>:"Add State(s) to Queue__JKI_lib_State_Machine.vi"("State(s) in (\"\")"=w373) -> ("States Out"=w372:string)  [unwired: 14 in]
            }
          }
        }
        n112 = call "uuid.vi"() -> ("UUID"=w66:string)  [unwired: 11 in]
        n113 = call "CSM - Wait and Send Message for Reply.vi"("State"="API: Test State A", "Arguments (\"\")"=w66, "Target Module"=w68, "Error In (No Error)"=w30) -> ("error out"=w28:errorcluster)  [unwired: 8 in, 3 out]
        n114 = call "uuid.vi"() -> ("UUID"=w65:string)  [unwired: 11 in]
        n115 = call "CSM - Wait and Send Message for Reply.vi"("State"="API: Test State B", "Arguments (\"\")"=w65, "Target Module"=w67, "Error In (No Error)"=w28) -> ("error out"=w27:errorcluster)  [unwired: 8 in, 3 out]
        n116 = call "Stall Data Flow.vim"("value in"=w27, "milliseconds to wait"=u32 100) -> ("value out"=w55:errorcluster)  [unwired: 1 out]
        n117 = call "CSM Get Module Attribute.vim"("CSM Name"=w29, "Attribute"=w50, "Default Value (Empty Variant)"=0 ("y"), "Error In"=w55) -> ("Found"=w54:bool, "Value"=w53:i32, "error out"=w44:errorcluster)  [unwired: 7 in, 2 out]
        n118 = call "Package Error Info.vi"("error in"=w36, "String in"=w32) -> ("packed error info out"=w40:string, "error status"=w41:bool)  [unwired: 8 in]
        n119 = flat-sequence {
          tunnel: w29 -> [w75]
          tunnel: w50 -> [w74]
          tunnel: w44 -> [w73]
          tunnel: [w71] -> w43
          tunnel: w43 -> [w81]
          tunnel: w29 -> [w78]
          tunnel: [w77] -> w36
          frame #0 {
            n120 = call "CSM - Delete Module Attribute.vi"("CSM Name"=w75, "Attribute"=w74) -> ("error out"=w72:errorcluster)  [unwired: 10 in, 3 out]
            n121 = Merge Errors(w73, w72) -> (w71:errorcluster)
          }
          frame #1 {
            n122 = call "CSM - Wait and Send Message for Reply.vi"("State"="Macro: Exit", "Target Module"=w78) -> ("error out"=w80:errorcluster)  [unwired: 10 in, 3 out]
            n123 = call <vilib>:"Clear Errors.vi"("error in (no error)"=w80) -> ("error out"=w76:errorcluster)  [unwired: 5 in, 1 out]
            n124 = Merge Errors(w81, w76) -> (w77:errorcluster)
          }
        }
        n125 = Equal?(x=w53, y=2) -> (x = y?=w51:bool)
        n126 = call-dynamic "failIf.vi"("message (\"\")"=w40, "fail"=w41, "TestCase in"=w39) -> ("error out"=w37:errorcluster, "TestCase out"=w38:refnum<class "testcase-CSMBroadcast.lvclass">)  [unwired: 7 in]
        n127 = And(x=w54, y=w51) -> (x .and. y?=w49:bool)
        n128 = call-dynamic "passIf.vi"("error in (no error)"=w37, "message (\"\")"=w32, "pass"=w49, "TestCase in"=w38) -> ("error out"=w47:errorcluster, "TestCase out"=w48:refnum<class "testcase-CSMBroadcast.lvclass">)  [unwired: 6 in]
      }
      n129 = flat-sequence {
        tunnel: w17 -> [w26]
        tunnel: [w25] -> w15
        tunnel: w18 -> [w23]
        tunnel: [w23] -> w16
        frame #0 {
          n130 = call "CSM - Drop Broadcast Registry.vi"() -> ("error out"=w24:errorcluster)  [unwired: 15 in]
          n131 = Merge Errors(w26, w24) -> (w25:errorcluster)
        }
      }
    }
    frame Disabled {
      # "skip test result while test is under development"
      n132 = call <vilib>:"skip.vi"("error in (no error)"=w374, "TestCase in"=w377) -> ("error out"=w376:errorcluster, "TestCase out"=w375:refnum<class "testcase-CSMBroadcast.lvclass">)  [unwired: 8 in]
    }
  }
  "error out" <- w4
  "TestCase out" <- w2
